vi "Test_MergeErrorsPublication_ErrorArray_1stErrorMerged.vi"(8 "error in (no error)":errorcluster, 11 "TestCase in":refnum<class "TestPublicationPolicy.lvclass">) -> (0 "error out":errorcluster, 3 "TestCase out":refnum<class "TestPublicationPolicy.lvclass">)   [LabVIEW 2017, in "TestPublicationPolicy.lvclass"]
uses:
  TestPublicationPolicy.lvclass
  gpm_packages/@cs/mva-core/Source/IMediator/MutexedPublishRequest/MutexedPublishRequest.lvclass
  gpm_packages/@cs/mva-core/Source/IMediator/IPublicationPolicy/IPublicationPolicy.lvclass
  gpm_packages/@cs/mva-core/Source/PublicationPolicy/MergeErrorsPublication/MergeErrorsPublication.lvclass
  gpm_packages/@cs/transport/Source/Concrete/NotifierTransport/NotifierTransport.lvclass
  C:/Git/mva-framework/Source/Framework/IMediator/IPublicationPolicy/IPublicationPolicy.lvclass
  C:/Git/mva-framework/gpm_packages/@cs/transport/Source/ITransport/ITransport.lvclass
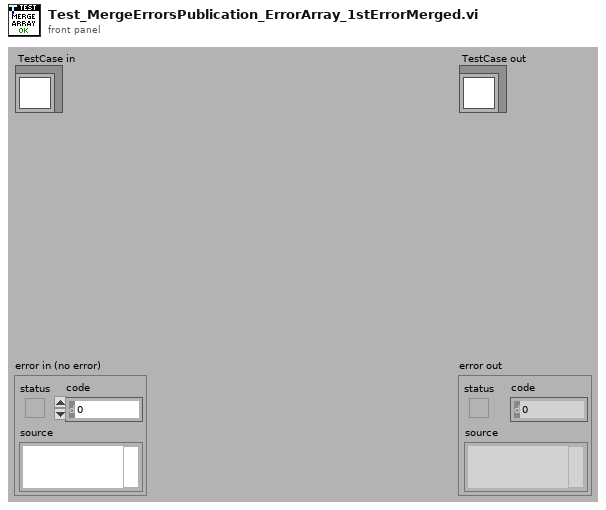
[diagram p1: front panel]
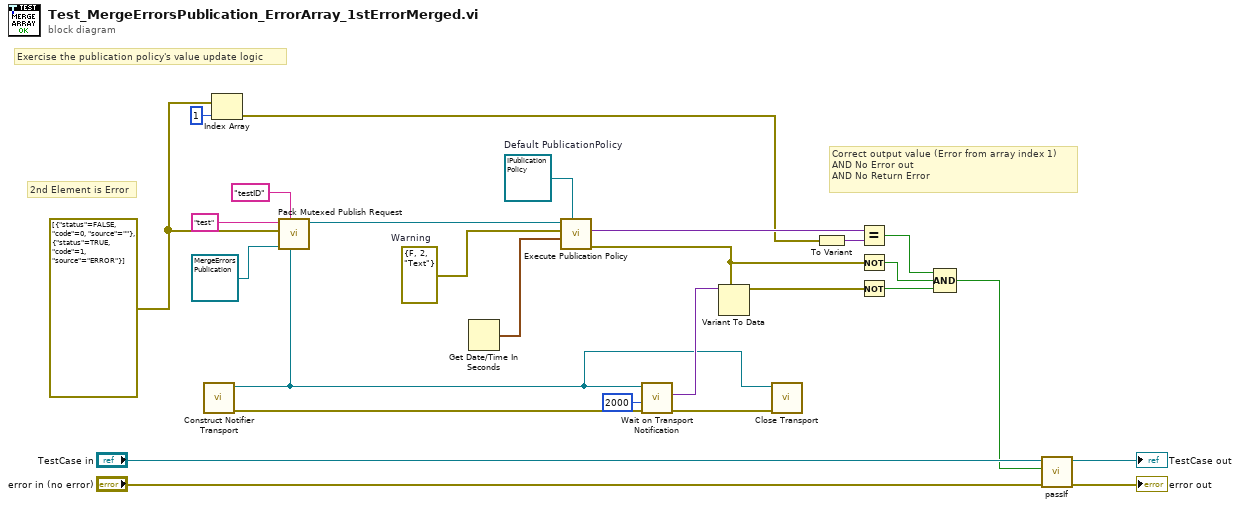
[diagram p0: block diagram]
diagram:
  w5 = errorcluster[] [{"status"=FALSE, "code"=0, "source"=""}, {"status"=TRUE, "code"=1, "source"="ERROR"}] ("error constant")
  w20 = refnum<class "IPublicationPolicy.lvclass"> refnum  # Default PublicationPolicy
  w6 = errorcluster {"status"=FALSE, "code"=2, "source"="Text"}  # Warning
  # "2nd Element is Error"
  # "Correct output value (Error from array index 1)\nAND No Error out\nAND No Return Error"
  # "Exercise the publication policy's value update logic"
  n1 = call "Construct Notifier Transport.vi"() -> ("error out"=w17:errorcluster, "NotifierTransport"=w2:refnum<class "NotifierTransport.lvclass">)  [unwired: 10 in]
  n2 = Index Array(array=w5, index=1) -> (element=w3:errorcluster)
  n3 = call "Pack Mutexed Publish Request.vi"("Return Error Transport"=w2, "Publisher ID"="testID", "error in (no error)"=refnum<class "MergeErrorsPublication.lvclass"> refnum ("PublicationPolicy.lvlib:MergeErrorsPublication.lvclass"), "Datum Value or Type"=w5, "Datum Name"="test") -> ("MutexedPublishRequest Out"=w22:refnum<class "MutexedPublishRequest.lvclass">)  [unwired: 5 in, 1 out]
  n4 = Get Date/Time In Seconds() -> (seconds since 1Jan1904=w23:timestamp)
  n5 = call-dynamic "Execute Publication Policy.vi"("Default PublicationPolicy"=w20, "Last Publish Time"=w23, "Last Published Value"=w6, "MutexedPublishRequest"=w22) -> ("error out (Reject Publication)"=w9:errorcluster, "Value to Publish"=w14:variant)  [unwired: 5 in, 1 out]
  n6 = call "Wait on Transport Notification.vi"("error in (no error)"=w17, "Timeout In ms (-1)"=2000, "NotifierTransport"=w2) -> ("error out"=w1:errorcluster, "Data"=w15:variant)  [unwired: 6 in, 1 out]
  n7 = Variant To Data(type=w9, Variant=w15) -> (data=w12:errorcluster)  [unwired: 1 in, 1 out]
  n8 = call-dynamic "Close Transport.vi"("error in (no error)"=w1, "NotifierTransport"=w2) -> ()  [unwired: 9 in, 1 out]
  n9 = To Variant(anything=w3) -> (Variant=w13:variant)
  n10 = Equal?(x=w14, y=w13) -> (x = y?=w11:bool)
  n11 = Not(x=w9) -> (.not. x?=w8:bool)
  n12 = Not(x=w12) -> (.not. x?=w10:bool)
  n13 = Compound Arithmetic op=AND(w11, w8, w10) -> (w7:bool)
  n14 = call-dynamic "passIf.vi"("error in (no error)"="error in (no error)", "pass"=w7, "TestCase in"="TestCase in") -> ("error out"=→"error out":errorcluster, "TestCase out"=→"TestCase out":refnum<class "TestPublicationPolicy.lvclass">)  [unwired: 7 in]
